vi "ChangeFileExtension.vi"(8 "ErrorIn":errorcluster, 10 "NewExtension":string, 11 "OldPath":path) -> (0 "ErrorOut":errorcluster, 3 "NewPath":path)   [LabVIEW 2017]
doc: "A convenience VI simplifying the process of changing a file extension.\n\ninfo@becker-hickl.com"
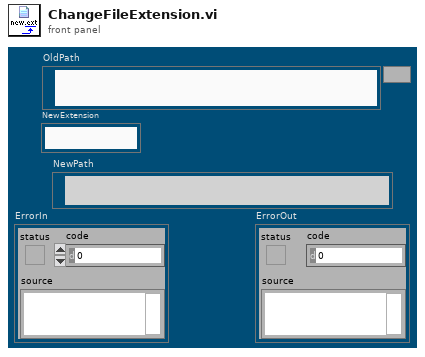
[diagram p1: front panel]
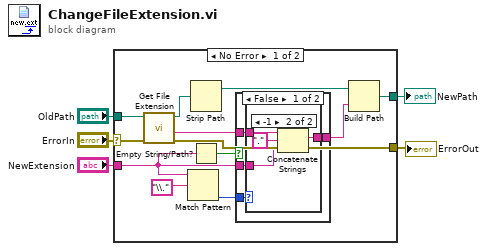
[diagram p0: block diagram]
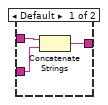
[diagram p2: hidden frame]
diagram:
  n1 = case shown="No Error" "ErrorIn" {
    selector: "ErrorIn" -> [w10 w31]
    tunnel: "OldPath" -> [w11 w30]
    tunnel: [w17 w30] -> w4
    tunnel: "NewExtension" -> [w12 _]
    tunnel: [w6 w31] -> w2
    frame No Error {
      n2 = call <vilib>:"Get File Extension.vi"("error in (no error)"=w10, "file"=w11) -> ("error out"=w6:errorcluster, "filename without extension"=w7:string, "dup file"=w9:path)  [unwired: 7 out]
      n3 = Match Pattern(string=w12, regular expression="\\." ("string")) -> (offset past match=w14:i32)  [unwired: 4 out]
      n4 = Strip Path(path=w9) -> (stripped path=w8:path)  [unwired: 1 out]
      n5 = Empty String/Path?(string/path=w12) -> (empty?=w13:bool)
      n6 = case shown="False" w13 {
        tunnel: [w21 w29] -> w16
        tunnel: w7 -> [w20 w29]
        tunnel: w12 -> [w19 _]
        tunnel: w14 -> [w18 _]
        frame False {
          n7 = case shown="-1" w18 {
            tunnel: [w22 w28] -> w21
            tunnel: w20 -> [w24 w27]
            tunnel: w19 -> [w23 w25]
            frame Default {
              n8 = Concatenate Strings(w24, w23) -> (w22:string)
            }
            frame -1 {
              n9 = Concatenate Strings(w27, "." ("string"), w25) -> (w28:string)
            }
          }
        }
        frame True {
        }
      }
      n10 = Build Path(base path=w8, name or relative path=w16) -> (appended path=w17:path)
    }
    frame Error {
    }
  }
  "NewPath" <- w4
  "ErrorOut" <- w2
